vi "addEdge.vi"(0 "reference":refnum<class "CallNode.lvclass">, 1 "egde":refnum<class "AbstractEdge.lvclass">, 2 "p1":T1 {"y" format="%.2f"; "x" format="%.2f"}, 3 "p2":T1 {"y" format="%.2f"; "x" format="%.2f"}, 5 "error in (no error)":errorcluster) -> (14 "reference out":refnum<class "CallNode.lvclass">, 15 "edgeHasEndNode":bool, 19 "error out":errorcluster)   [LabVIEW 2012, in "CallNode.lvclass"]
doc: "public boolean addEdge(Edge e, Point2D p1, Point2D p2)"
uses:
  <resource>/Framework/Providers/Open_GDS/UML/CallNode_class/CallNode.lvclass
  <resource>/Framework/Providers/Open_GDS/UML/AbstractEdge_class/AbstractEdge.lvclass
  <resource>/Framework/Providers/Open_GDS/UML/General/Point/Point Point2D.ctl
  <resource>/Framework/Providers/Open_GDS/UML/ImplicitParameterNode_class/ImplicitParameterNode.lvclass
  <resource>/Framework/Providers/Open_GDS/UML/SegmentedLineEdge_class/SegmentedLineEdge.lvclass
  <resource>/Framework/Providers/Open_GDS/UML/AbstractNode_class/AbstractNode.lvclass
  <resource>/Framework/Providers/Open_GDS/UML/RectangularNode_class/RectangularNode.lvclass
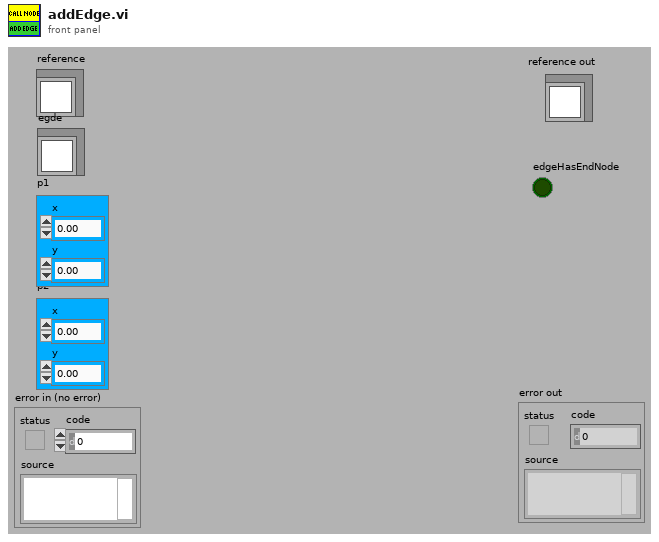
[diagram p1: front panel]
types:
  T1 = typedef "Point Point2D.ctl" = cluster{"x":dbl, "y":dbl}
  T2 = typedef "CallNode.lvclass/ObjectAttributes.ctl" = cluster{"Base class":T3, "objectCallNodeRef":refnum<class "AbstractNode.lvclass">, "signaled":bool, "openBottom":bool, "DEFAULT_WIDTH":i32, "DEFAULT_HEIGHT":i32, "CALL_YGAP":i32}
  T3 = typedef "RectangularNode.lvclass/ObjectAttributes.ctl" = cluster{"Base class":T4, "bounds":T5}
  T4 = typedef "AbstractNode.lvclass/ObjectAttributes.ctl" = cluster{"parent":refnum<class "AbstractNode.lvclass">, "children":refnum<class "AbstractNode.lvclass">[], "Hidden":bool}
  T5 = typedef "Rectangle Rectangle2D.ctl" = cluster{"x":dbl, "y":dbl, "width":dbl, "height":dbl}
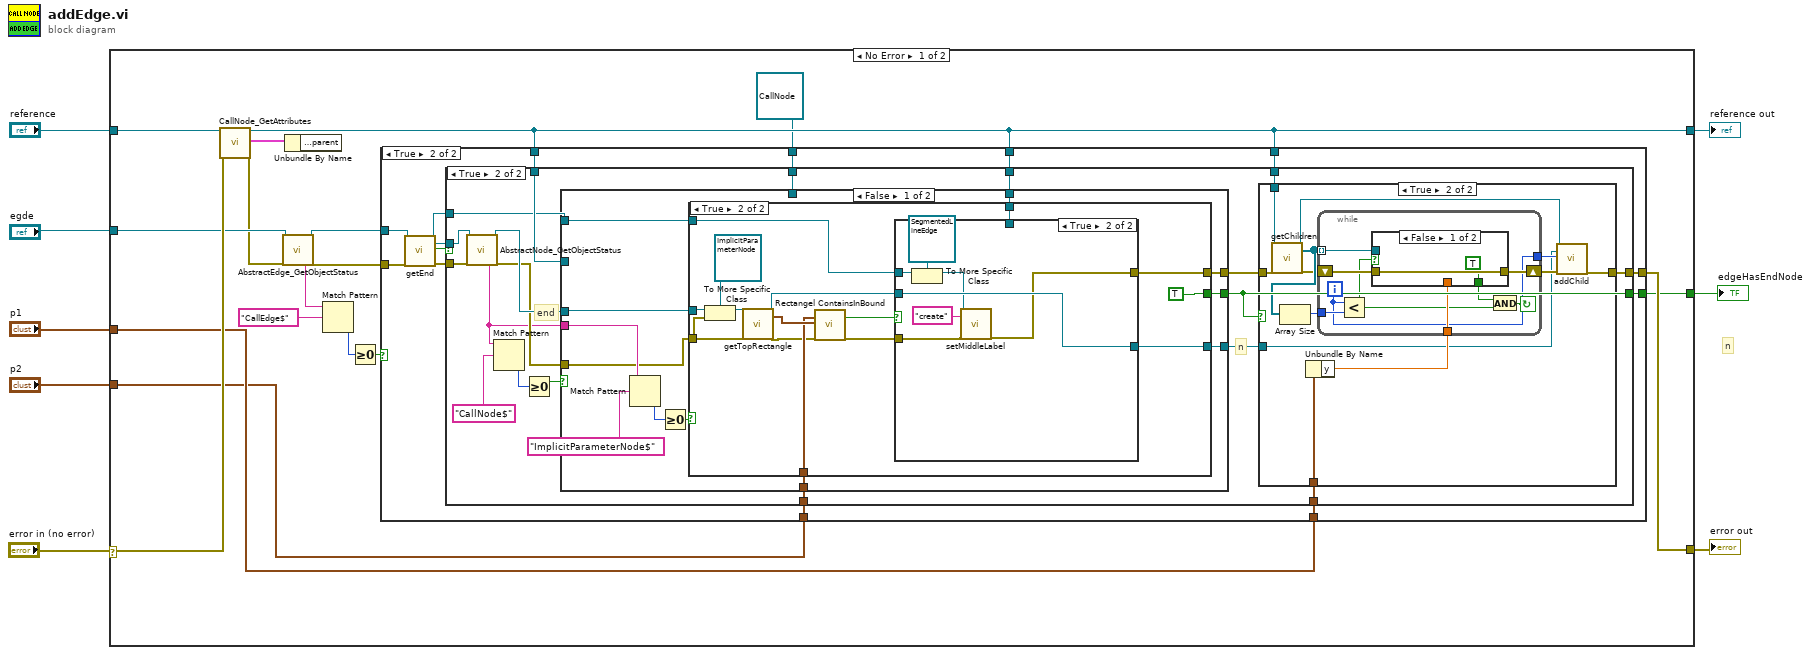
[diagram p0: block diagram]
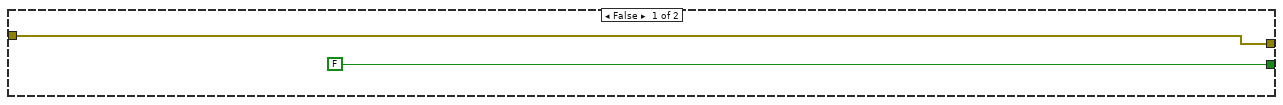
[diagram p2: hidden frame]
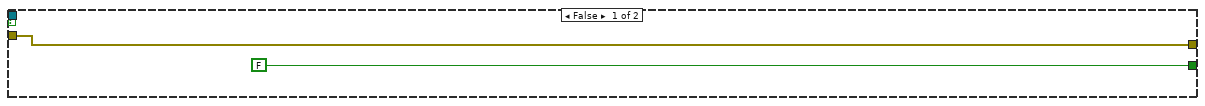
[diagram p3: hidden frame]
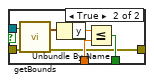
[diagram p5: hidden frame]
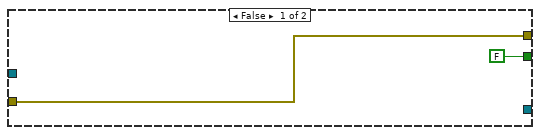
[diagram p6: hidden frame]
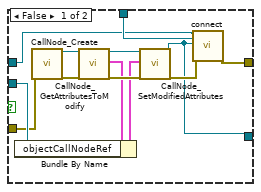
[diagram p7: hidden frame]
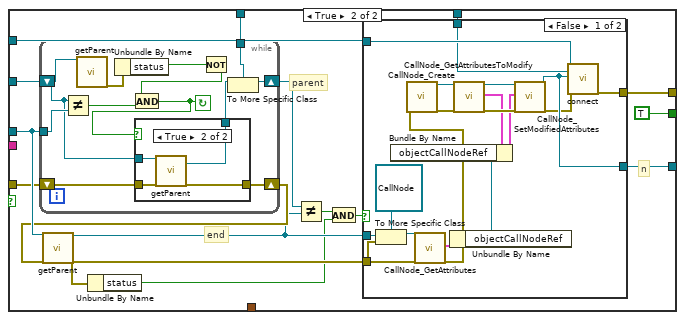
[diagram p8: hidden frame]
diagram:
  # "n"
  n1 = case shown="No Error" "error in (no error)" {
    selector: "error in (no error)" -> [w22 w197]
    tunnel: "reference" -> [w25 w198]
    tunnel: [w24 w197] -> w7
    tunnel: [w23 w198] -> w6
    tunnel: "egde" -> [w21 _]
    tunnel: [w20 _] -> w3
    tunnel: "p1" -> [w19 _]
    tunnel: "p2" -> [w18 _]
    frame No Error {
      n2 = call <resource>:"CallNode_GetAttributes.vi"("reference in"=w25, "error in (no error)"=w22) -> ("reference out"=w23:refnum<class "CallNode.lvclass">, "Attributes"=w17:T2, "error out"=w12:errorcluster)  [unwired: 15 out]
      n3 = call <resource>:"AbstractEdge_GetObjectStatus.vi"("reference in"=w21, "error in (no error)"=w12) -> ("Class name"=w16:string, "reference out"=w11:refnum<class "AbstractEdge.lvclass">, "error out"=w10:errorcluster)  [unwired: 15 out]
      n4 = Unbundle By Name(w17) -> ()  [unwired: 1 out]
      n5 = Match Pattern(string=w16, regular expression="CallEdge$") -> (offset past match=w14:i32)  [unwired: 4 out]
      n6 = Greater Or Equal To 0?(x=w14) -> (x >= 0?=w13:bool)
      n7 = case shown="True" w13 {
        tunnel: [FALSE w41] -> w20
        tunnel: w11 -> [_ w40]
        tunnel: w10 -> [w26 w39]
        tunnel: w23 -> [_ w35]
        tunnel: w23 -> [_ w33]
        tunnel: w18 -> [_ w32]
        tunnel: w23 -> [_ w31]
        tunnel: w19 -> [_ w30]
        tunnel: [w26 w29] -> w24
        tunnel: refnum<class "CallNode.lvclass"> refnum ("reference out") -> [_ w28]
        frame False {
        }
        frame True {
          n8 = call-dynamic "getEnd.vi"("reference"=w40, "error in (no error)"=w39) -> ("reference out"=w34:refnum<class "AbstractEdge.lvclass">, "endNode"=w37:refnum<class "AbstractNode.lvclass">, "validNode"=w38:bool, "error out"=w36:errorcluster)  [unwired: 14 in]
          n9 = case shown="True" w38 {
            tunnel: [FALSE w50] -> w41
            tunnel: w37 -> [_ w62]
            tunnel: w36 -> [w42 w61]
            tunnel: w35 -> [_ w57]
            tunnel: w34 -> [_ w54]
            tunnel: w33 -> [_ w53]
            tunnel: w32 -> [_ w51]
            tunnel: w31 -> [_ w49]
            tunnel: w30 -> [_ w47]
            tunnel: [w42 w45] -> w29
            tunnel: w28 -> [_ w44]
            frame False {
            }
            frame True {
              # "n"
              # "end"
              n10 = call <resource>:"AbstractNode_GetObjectStatus.vi"("reference in"=w62, "error in (no error)"=w61) -> ("Class name"=w52:string, "reference out"=w56:refnum<class "AbstractNode.lvclass">, "error out"=w55:errorcluster)  [unwired: 15 out]
              n11 = Match Pattern(string=w52, regular expression="CallNode$") -> (offset past match=w60:i32)  [unwired: 4 out]
              n12 = Greater Or Equal To 0?(x=w60) -> (x >= 0?=w58:bool)
              n13 = case shown="False" w58 {
                tunnel: w57 -> [_ w158]
                tunnel: w56 -> [w100 w157]
                tunnel: w55 -> [w99 w154]
                tunnel: w54 -> [w96 w151]
                tunnel: w53 -> [w95 w150]
                tunnel: w52 -> [w103 _]
                tunnel: [w102 TRUE] -> w50
                tunnel: w51 -> [w98 _]
                tunnel: [w97 w148] -> w46
                tunnel: [w94 w146] -> w48
                tunnel: w44 -> [_ w145]
                frame False {
                  n14 = Match Pattern(string=w103, regular expression="ImplicitParameterNode$") -> (offset past match=w104:i32)  [unwired: 4 out]
                  n15 = Greater Or Equal To 0?(x=w104) -> (x >= 0?=w101:bool)
                  n16 = case shown="True" w101 {
                    tunnel: [FALSE TRUE] -> w102
                    tunnel: w100 -> [_ w110]
                    tunnel: w99 -> [w106 w111]
                    tunnel: w98 -> [_ w120]
                    tunnel: [_ w117] -> w97
                    tunnel: w96 -> [_ w115]
                    tunnel: w95 -> [_ w113]
                    tunnel: [w106 w112] -> w94
                    frame False {
                    }
                    frame True {
                      n17 = To More Specific Class(target class=refnum<class "ImplicitParameterNode.lvclass"> refnum ("reference"), reference=w110, error in=w111) -> (specific class reference=w108:refnum<class "ImplicitParameterNode.lvclass">)  [unwired: 1 out]
                      n18 = call-dynamic "getTopRectangle.vi"("reference"=w108, "error in (no error)"=w111) -> ("reference out"=w116:refnum<class "ImplicitParameterNode.lvclass">, "bounds"=w121:T5, "error out"=w119:errorcluster)  [unwired: 15 in]
                      n19 = call <resource>:"Rectangel ContainsInBound.vi"("point2D"=w120, "bounds"=w121, "error in (no error)"=w119) -> ("contains"=w118:bool, "error out"=w114:errorcluster)  [unwired: 1 in, 14 out]
                      n20 = case shown="True" w118 {
                        tunnel: [w124 w140] -> w117
                        tunnel: w116 -> [w129 w140]
                        tunnel: w115 -> [w125 w137]
                        tunnel: w114 -> [w128 w142]
                        tunnel: w113 -> [w126 _]
                        tunnel: [w123 w139] -> w112
                        frame False {
                          n21 = call <resource>:"CallNode_Create.vi"("error in (no error)"=w128) -> ("reference out"=w133:refnum<class "CallNode.lvclass">, "error out"=w132:errorcluster)  [unwired: 2 in, 15 out]
                          n22 = call <resource>:"CallNode_GetAttributesToModify.vi"("reference in"=w133, "error in (no error)"=w132) -> ("reference out"=w135:refnum<class "CallNode.lvclass">, "Attributes"=w130:T2, "error out"=w134:errorcluster)  [unwired: 1 in, 14 out]
                          n23 = Bundle By Name(cluster=w130, "objectCallNodeRef"=w129) -> (w131:T2)
                          n24 = call <resource>:"CallNode_SetModifiedAttributes.vi"("reference in"=w135, "Attributes"=w131, "error in (no error)"=w134) -> ("reference out"=w124:refnum<class "CallNode.lvclass">, "error out"=w127:errorcluster)  [unwired: 3 in, 12 out]
                          n25 = call-dynamic "connect.vi"("reference"=w125, "startNode"=w126, "endNode"=w124, "error in (no error)"=w127) -> ("error out"=w123:errorcluster)  [unwired: 14 in, 1 out]
                        }
                        frame True {
                          n26 = To More Specific Class(target class=refnum<class "SegmentedLineEdge.lvclass"> refnum ("reference"), reference=w137) -> (specific class reference=w136:refnum<class "SegmentedLineEdge.lvclass">)  [unwired: 1 in, 1 out]
                          n27 = call-dynamic "setMiddleLabel.vi"("reference"=w136, "middleLabel"="create", "error in (no error)"=w142) -> ("error out"=w139:errorcluster)  [unwired: 15 in, 1 out]
                        }
                      }
                    }
                  }
                }
                frame True {
                  # "parent"
                  # "end"
                  # "n"
                  n28 = while {
                    shift-right: [w183] -> w156
                    shift-left: w158 -> [w182]
                    tunnel: w157 -> [w190]
                    shift-right: [w186] -> w155
                    shift-left: w154 -> [w187]
                    tunnel: w145 -> [w184]
                    stop <- w188 continue-if-true
                    n29 = Not Equal?(x=w182, y=w190) -> (x != y?=w189:bool)
                    n30 = call-dynamic "getParent.vi"("reference"=w182) -> ("error out"=w181:errorcluster)  [unwired: 14 in, 4 out]
                    n31 = Unbundle By Name(w181) -> ("status"=w180:bool)
                    n32 = Not(x=w180) -> (.not. x?=w179:bool)
                    n33 = And(x=w179, y=w189) -> (x .and. y?=w188:bool)
                    n34 = case shown="True" w188 {
                      tunnel: w182 -> [w192 w196]
                      tunnel: [w192 w195] -> w185
                      tunnel: w187 -> [w191 w194]
                      tunnel: [w191 w193] -> w186
                      frame False {
                      }
                      frame True {
                        n35 = call-dynamic "getParent.vi"("reference"=w196, "error in (no error)"=w194) -> ("parentNode"=w195:refnum<class "AbstractNode.lvclass">, "error out"=w193:errorcluster)  [unwired: 13 in, 3 out]
                      }
                    }
                    n36 = To More Specific Class(target class=w184, reference=w185) -> (specific class reference=w183:refnum<class "CallNode.lvclass">)  [unwired: 1 in, 1 out]
                  }
                  n37 = call-dynamic "getParent.vi"("reference"=w157, "error in (no error)"=w155) -> ("reference out"=w149:refnum<class "AbstractNode.lvclass">, "error out"=w144:errorcluster)  [unwired: 13 in, 3 out]
                  n38 = Unbundle By Name(w144) -> ("status"=w143:bool)
                  n39 = Not Equal?(x=w156, y=w149) -> (x != y?=w153:bool)
                  n40 = And(x=w153, y=w143) -> (x .and. y?=w152:bool)
                  n41 = case shown="False" w152 {
                    tunnel: w149 -> [w161 w178]
                    tunnel: [w167 w178] -> w148
                    tunnel: w151 -> [w169 _]
                    tunnel: w150 -> [w168 _]
                    tunnel: w144 -> [w162 w177]
                    tunnel: [w163 w177] -> w146
                    frame False {
                      n42 = To More Specific Class(target class=refnum<class "CallNode.lvclass"> refnum ("reference out"), reference=w161, error in=w162) -> (specific class reference=w160:refnum<class "CallNode.lvclass">)  [unwired: 1 out]
                      n43 = call <resource>:"CallNode_GetAttributes.vi"("reference in"=w160, "error in (no error)"=w162) -> ("Attributes"=w176:T2, "error out"=w165:errorcluster)  [unwired: 16 out]
                      n44 = call <resource>:"CallNode_Create.vi"("error in (no error)"=w165) -> ("reference out"=w173:refnum<class "CallNode.lvclass">, "error out"=w172:errorcluster)  [unwired: 2 in, 15 out]
                      n45 = Unbundle By Name(w176) -> ("objectCallNodeRef"=w166:refnum<class "AbstractNode.lvclass">)
                      n46 = call <resource>:"CallNode_GetAttributesToModify.vi"("reference in"=w173, "error in (no error)"=w172) -> ("reference out"=w175:refnum<class "CallNode.lvclass">, "Attributes"=w170:T2, "error out"=w174:errorcluster)  [unwired: 1 in, 14 out]
                      n47 = Bundle By Name(cluster=w170, "objectCallNodeRef"=w166) -> (w171:T2)
                      n48 = call <resource>:"CallNode_SetModifiedAttributes.vi"("reference in"=w175, "Attributes"=w171, "error in (no error)"=w174) -> ("reference out"=w167:refnum<class "CallNode.lvclass">, "error out"=w164:errorcluster)  [unwired: 3 in, 12 out]
                      n49 = call-dynamic "connect.vi"("reference"=w169, "startNode"=w168, "endNode"=w167, "error in (no error)"=w164) -> ("error out"=w163:errorcluster)  [unwired: 14 in, 1 out]
                    }
                    frame True {
                    }
                  }
                }
              }
              n50 = case shown="True" w50 {
                tunnel: w49 -> [_ w75]
                tunnel: w48 -> [w63 w74]
                tunnel: w47 -> [_ w70]
                tunnel: w46 -> [_ w65]
                tunnel: [w63 w64] -> w45
                frame False {
                }
                frame True {
                  n51 = call-dynamic "getChildren.vi"("reference"=w75, "error in (no error)"=w74) -> ("reference out"=w67:refnum<class "CallNode.lvclass">, "children"=w73:refnum<class "AbstractNode.lvclass">[], "error out"=w71:errorcluster)  [unwired: 14 in, 1 out]
                  n52 = Array Size(array=w73) -> (size(s)=w72:i32)
                  n53 = Unbundle By Name(w70) -> ("y"=w69:dbl)
                  n54 = while {
                    shift-right: [w78] -> w68
                    shift-left: w71 -> [w83]
                    tunnel: w73 -> [w82] mode=indexing
                    tunnel: w72 -> [w84]
                    tunnel: w69 -> [w81]
                    tunnel: [w77] -> w66
                    i -> [w77]
                    stop <- w79 continue-if-true
                    n55 = Less?(x=w77, y=w84) -> (x < y?=w76:bool)
                    n56 = case shown="False" w76 {
                      tunnel: w83 -> [w86 w93]
                      tunnel: w82 -> [_ w92]
                      tunnel: w81 -> [_ w89]
                      tunnel: [TRUE w88] -> w80
                      tunnel: [w86 w87] -> w78
                      frame False {
                      }
                      frame True {
                        n57 = call-dynamic "getBounds.vi"("reference"=w92, "error in (no error)"=w93) -> ("bounds"=w91:T5, "error out"=w87:errorcluster)  [unwired: 15 in, 1 out]
                        n58 = Unbundle By Name(w91) -> ("y"=w90:dbl)
                        n59 = Less Or Equal?(x=w90, y=w89) -> (x <= y?=w88:bool)
                      }
                    }
                    n60 = And(x=w80, y=w76) -> (x .and. y?=w79:bool)
                  }
                  n61 = call-dynamic "addChild.vi"("reference"=w67, "node"=w65, "index(last)"=w66, "error in (no error)"=w68) -> ("error out"=w64:errorcluster)  [unwired: 14 in, 1 out]
                }
              }
            }
          }
        }
      }
    }
    frame Error {
    }
  }
  "reference out" <- w6
  "error out" <- w7
  "edgeHasEndNode" <- w3
